vi "TCP_M 서버장난감.vi"() -> ()   [LabVIEW 2018]
uses:
  labview study/TypeDefine/Server Status.ctl
panel:
  out "데이터 출력":string
  out "Current Data":dbl
  in  "정지":bool
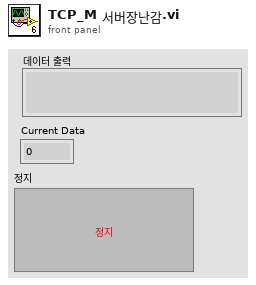
[diagram p1: front panel]
types:
  T1 = typedef "Server Status.ctl" = enum16{"초기화", "Listen and Connect", "Send Data", "Stop"}
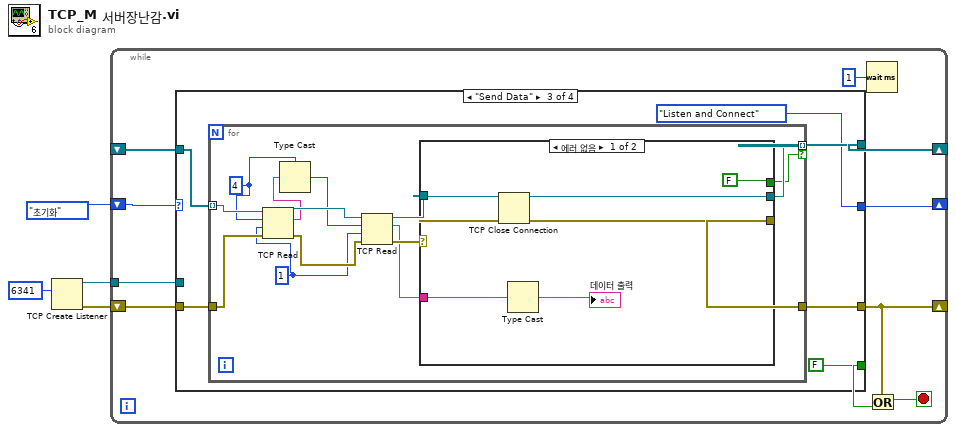
[diagram p0: block diagram]
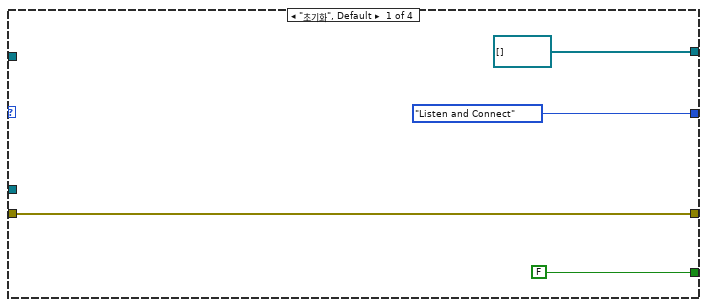
[diagram p2: hidden frame]
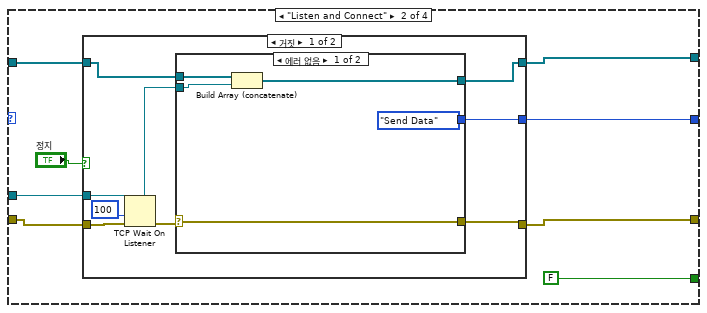
[diagram p3: hidden frame]
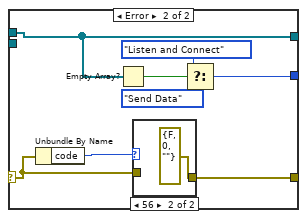
[diagram p4: hidden frame]
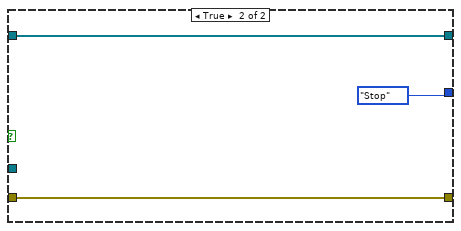
[diagram p6: hidden frame]
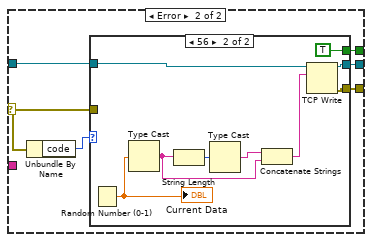
[diagram p7: hidden frame]
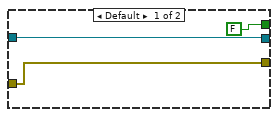
[diagram p8: hidden frame]
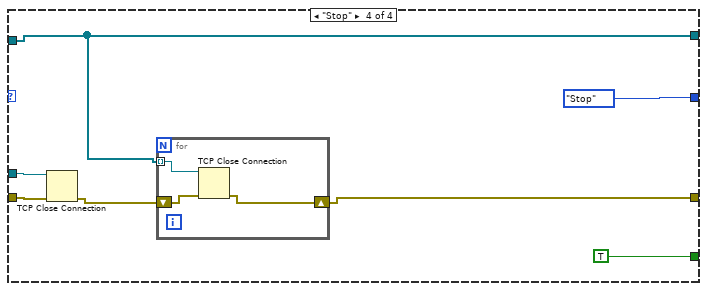
[diagram p9: hidden frame]
diagram:
  n1 = TCP Create Listener(10:u16 6341 ("포트")) -> (0:w3:errorcluster, 3:w2:refnum<k5>)  [unwired: 4 in, 1 out]
  n2 = while {
    shift-right: [w13] -> _
    shift-left: Server_Status."초기화" ("열거형") -> [w14]
    shift-right: [w9] -> _
    shift-left: w3 -> [w11]
    tunnel: w2 -> [w12]
    shift-right: [w6] -> _
    shift-left: _ -> [w7]
    stop <- w8 stop-if-true
    n3 = case shown="\"Send Data\"" w14 {
      tunnel: [Server_Status."Listen and Connect" ("열거형") w20 Server_Status."Listen and Connect" ("열거형") Server_Status."Stop" ("열거형")] -> w13
      tunnel: w12 -> [_ w23 _ w105]
      tunnel: [w17 w21 w56 w101] -> w9
      tunnel: w11 -> [w17 w22 w59 w104]
      tunnel: [FALSE FALSE FALSE TRUE] -> w10
      tunnel: w7 -> [_ w25 w58 w103]
      tunnel: [refnum<k5>[] [] w24 w57 w103] -> w6
      frame "초기화", Default {
      }
      frame "Listen and Connect" {
        n4 = case shown="거짓" "정지" {
          tunnel: [w29 w53] -> w24
          tunnel: w25 -> [w30 w53]
          tunnel: w23 -> [w35 _]
          tunnel: [w31 w52] -> w21
          tunnel: w22 -> [w34 w52]
          tunnel: [w27 Server_Status."Stop" ("열거형")] -> w20
          frame False {
            n5 = TCP Wait On Listener(8:w34, 9:100 ("타임아웃 ms (계속 기다림: -1)"), 11:w35) -> (0:w32:errorcluster, 4:w28:refnum<k5>)  [unwired: 1 in, 3 out]
            n6 = case shown="에러 없음" w32 {
              selector: w32 -> [w40 w47]
              tunnel: [w40 w46] -> w31
              tunnel: w30 -> [w39 w43]
              tunnel: [w38 w43] -> w29
              tunnel: w28 -> [w37 _]
              tunnel: [Server_Status."Send Data" ("열거형") w44] -> w27
              frame No Error {
                n7 = Build Array (concatenate)(w39, w37) -> (w38:refnum<k5>[])
              }
              frame Error {
                n8 = Unbundle By Name(w47) -> ("code"=w48:i32)
                n9 = Empty Array?(array=w43) -> (empty?=w45:bool)
                n10 = case shown="56" w48 {
                  tunnel: w47 -> [w49 _]
                  tunnel: [w49 errorcluster {"status"=FALSE, "code"=0, "source"=""} ("에러 상수")] -> w46
                  frame Default {
                  }
                  frame 56 {
                  }
                }
                n11 = Select(t=Server_Status."Listen and Connect" ("열거형"), s=w45, f=Server_Status."Send Data" ("열거형")) -> (s? t:f=w44:T1)
              }
            }
          }
          frame True {
          }
        }
      }
      frame "Send Data" {
        n12 = for {
          tunnel: w59 -> [w66]
          tunnel: w58 -> [w68] mode=indexing
          tunnel: [w71] -> w57 mode=indexing if=w69
          tunnel: [w70] -> w56
          w64 = 1 ("타임아웃 ms (25000)")
          w62 = 4 ("읽을 바이트")
          n13 = TCP Read(connection ID=w68, bytes to read=w62, error in (no error)=w66, 9:w64) -> (connection ID out=w67:refnum<k5>, data out=w63:string, error out=w65:errorcluster)  [unwired: 1 in]
          n14 = Type Cast(type=w62, x=w63) -> (*(type *) &x=w61:i32)
          n15 = TCP Read(connection ID=w67, bytes to read=w61, error in (no error)=w65, 9:w64) -> (connection ID out=w72:refnum<k5>, data out=w60:string, error out=w73:errorcluster)  [unwired: 1 in]
          n16 = case shown="에러 없음" w73 {
            selector: w73 -> [w79 w86]
            tunnel: w72 -> [w80 w84]
            tunnel: [w77 w83] -> w71
            tunnel: [w78 w82] -> w70
            tunnel: [FALSE w81] -> w69
            tunnel: w60 -> [w75 _]
            frame No Error {
              n17 = TCP Close Connection(connection ID=w80, error in (no error)=w79) -> (connection ID out=w77:refnum<k5>, error out=w78:errorcluster)  [unwired: 1 in]
              n18 = Type Cast(x=w75) -> (*(type *) &x=→"데이터 출력":string)  [unwired: 1 in]
            }
            frame Error {
              n19 = Unbundle By Name(w86) -> ("code"=w85:i32)
              n20 = case shown="56" w85 {
                tunnel: w86 -> [w89 _]
                tunnel: w84 -> [w88 w98]
                tunnel: [w88 w92] -> w83
                tunnel: [w89 w91] -> w82
                tunnel: [FALSE TRUE] -> w81
                frame Default {
                }
                frame 56 {
                  n21 = Random Number (0-1)() -> (number: 0 to 1=w97:dbl)
                  "Current Data" <- w97
                  n22 = Type Cast(x=w97) -> (*(type *) &x=w94:string)  [unwired: 1 in]
                  n23 = String Length(string=w94) -> (length=w96:i32)
                  n24 = Type Cast(x=w96) -> (*(type *) &x=w95:string)  [unwired: 1 in]
                  n25 = Concatenate Strings(w95, w94) -> (w93:string)
                  n26 = TCP Write(connection ID=w98, data in=w93) -> (connection ID out=w92:refnum<k5>, error out=w91:errorcluster)  [unwired: 2 in, 1 out]
                }
              }
            }
          }
        }
      }
      frame "Stop" {
        n27 = TCP Close Connection(connection ID=w105, error in (no error)=w104) -> (error out=w102:errorcluster)  [unwired: 1 in, 1 out]
        n28 = for {
          tunnel: w103 -> [w106] mode=indexing
          shift-right: [w107] -> w101
          shift-left: w102 -> [w108]
          n29 = TCP Close Connection(connection ID=w106, error in (no error)=w108) -> (error out=w107:errorcluster)  [unwired: 1 in, 1 out]
        }
      }
    }
    n30 = Wait (ms)(milliseconds to wait=u32 1 ("대기 시간 (ms)")) -> ()  [unwired: 1 out]
    n31 = Or(x=w9, y=w10) -> (x .or. y?=w8:bool)
  }
